vi "NI VeriStand - FPGA PWM Out.vi"(9 "_Low Time":u32, 11 "_High Time":u32) -> (3 "Output":bool)   [LabVIEW 2020, in "NI_VS FPGA Support.lvlib"]
uses:
  <vilib>/NI VeriStand/FPGA/NI_VS FPGA Support.lvlib
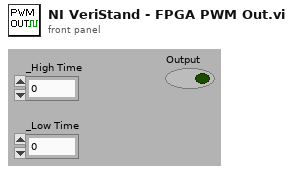
[diagram p1: front panel]
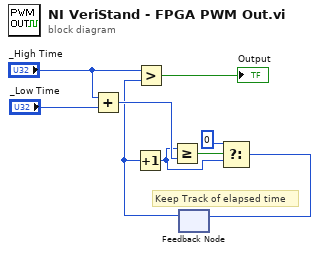
[diagram p0: block diagram]
diagram:
  # "Keep Track of elapsed time"
  n1 = Add(x="_High Time", y="_Low Time") -> (x+y=w8:u32)
  n2 = feedback #1() -> (w1:u32)  [unwired: 1 out]
  n3 = Increment(x=w1) -> (x+1=w5:u32)
  n4 = Greater?(x="_High Time", y=w1) -> (0:→"Output":bool)
  n5 = Greater Or Equal?(x=w5, y=w8) -> (x >= y?=w4:bool)
  n6 = Select(t=u32 0, s=w4, f=w5) -> (s? t:f=w2:u32)
  n7 = feedback-in #1(w2) -> ()
